vi "file_open_example.vi"() -> ()   [LabVIEW 2016]
panel:
  in  "operation (0:open)":T1(ring)
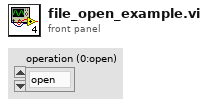
[diagram p1: front panel]
types:
  T1 = enum16{"open", "replace", "create", "open or create", "replace or create", "replace or create with confirmation"}
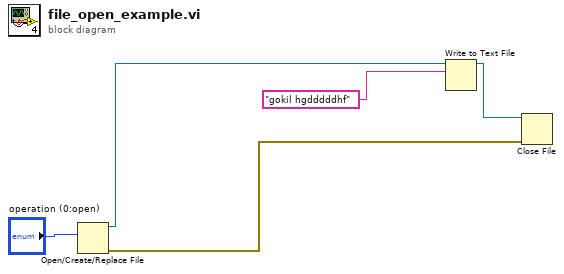
[diagram p0: block diagram]
diagram:
  n1 = Open/Create/Replace File(operation (0:open)="operation (0:open)") -> (refnum out=w4:refnum<file>, error out=w3:errorcluster)  [unwired: 5 in, 1 out]
  n2 = Write to Text File(file (use dialog)=w4, text="gokil hgdddddhf") -> (refnum out=w2:refnum<file>)  [unwired: 2 in, 2 out]
  n3 = Close File(refnum=w2, error in=w3) -> ()  [unwired: 2 out]
